vi "testClassA.vi"(8 "error in (no error)":errorcluster caption="Fehler (Eingang, kein Fehler)", 11 "test Eingang":refnum<class "test.lvclass"> caption="DNL_LabVIEW Object in") -> (0 "error out":errorcluster caption="Fehler (Ausgang)", 2 "Numerisch":dbl, 3 "test Ausgang":refnum<class "test.lvclass"> caption="DNL_LabVIEW Object out")   [LabVIEW 2013, in "test.lvclass"]
uses:
  test.lvclass
  test.lvclass/test.ctl
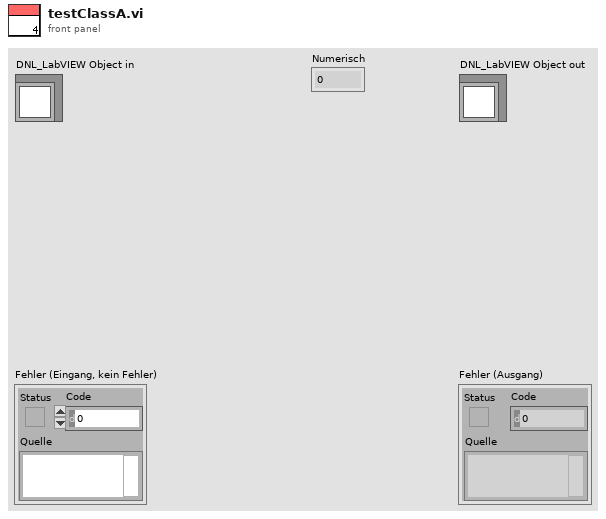
[diagram p1: front panel]
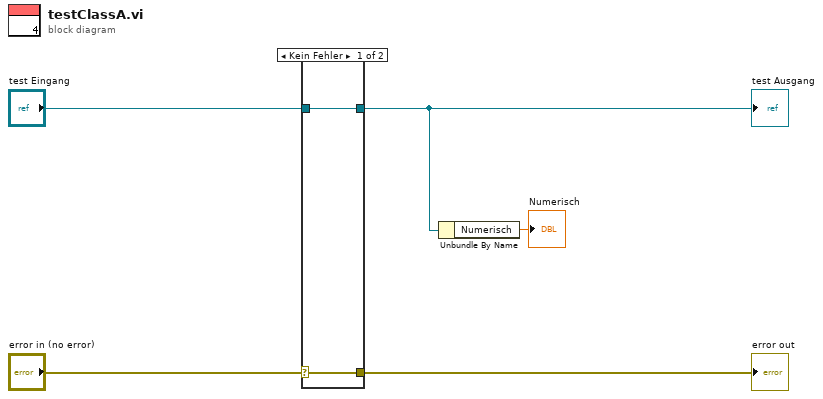
[diagram p0: block diagram]
diagram:
  n1 = case shown="Kein Fehler" "error in (no error)" {
    selector: "error in (no error)" -> [w7 w9]
    tunnel: [w7 w9] -> w4
    tunnel: [w6 w8] -> w2
    tunnel: "test Eingang" -> [w6 w8]
    frame No Error {
    }
    frame Error {
    }
  }
  "error out" <- w4
  "test Ausgang" <- w2
  n2 = Unbundle By Name(w2) -> ("Numerisch"=→"Numerisch":dbl)
